vi "NATS Async Monitor.vi"(6 "stop":refnum<notifier>, 8 "error in":errorcluster, 9 "message queue":refnum<queue>, 10 "request queue":refnum<queue>, 11 "nats connection in":T1={"connection ID"=refnum, "server INFO"="", "timeout ms"=5000, "verbose?"=FALSE, "server headers?"=FALSE, "client headers?"=FALSE}) -> (0 "error out":errorcluster)   [LabVIEW 2023, in "NATS Core.lvlib"]
doc: "Reads a message from the NATS server."
uses:
  NATS Core.lvlib
  Controls/nats connection.ctl
  Controls/request queue.ctl
  Controls/nats message.ctl
  Controls/msg type.ctl
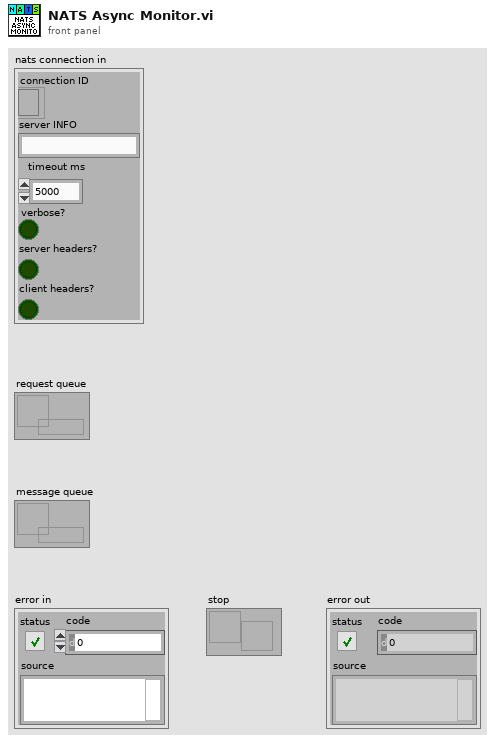
[diagram p1: front panel]
types:
  T1 = typedef "NATS Core.lvlib/nats connection.ctl" = cluster{"connection ID":refnum<k5>, "server INFO":string, "timeout ms":i32, "verbose?":bool, "server headers?":bool, "client headers?":bool}
  T2 = typedef "request queue.ctl" = cluster{"reply subject":string, "request queue":refnum<queue>}
  T3 = typedef "NATS Core.lvlib/nats message.ctl" = cluster{"subject":string, "payload":string, "sub id":string, "reply-to":string, "headers":string, "type":T4, "received":timestamp}
  T4 = typedef "NATS Core.lvlib/msg type.ctl" = enum16{"Undefined", "MSG", "HMSG", "+OK", "PING", "PONG", "-ERR", "INFO"}
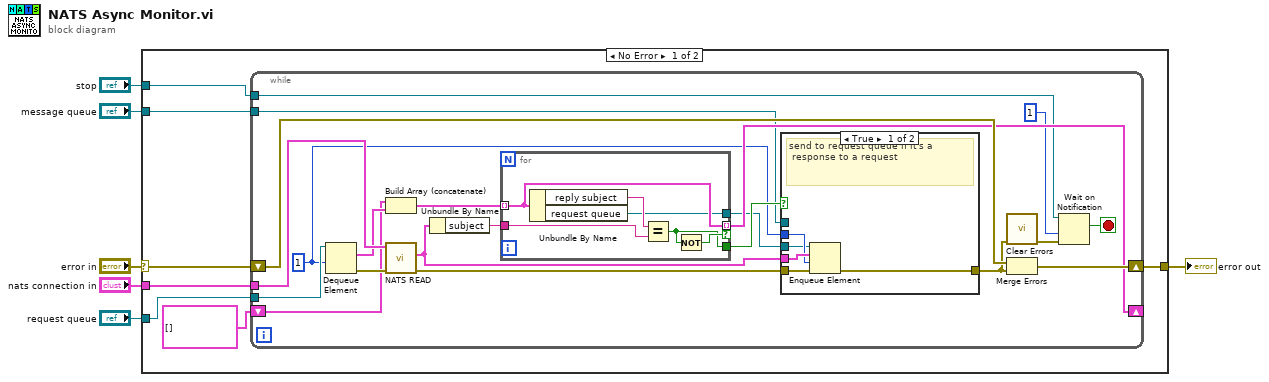
[diagram p0: block diagram]
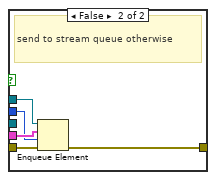
[diagram p2: hidden frame]
diagram:
  n1 = case shown="No Error" "error in" {
    selector: "error in" -> [w12 w51]
    tunnel: "nats connection in" -> [w11 _]
    tunnel: [w13 w51] -> w5
    tunnel: "request queue" -> [w10 _]
    tunnel: "message queue" -> [w8 _]
    tunnel: "stop" -> [w7 _]
    frame No Error {
      n2 = while {
        tunnel: w11 -> [w30]
        tunnel: w10 -> [w29]
        shift-right: [w24] -> _
        shift-left: T2[] [] -> [w27]
        tunnel: w8 -> [w20]
        tunnel: w7 -> [w17]
        shift-right: [w31] -> w13
        shift-left: w12 -> [w32]
        stop <- w16 stop-if-true
        w21 = 1 ("timeout in ms (-1)")
        n3 = Dequeue Element(queue=w29, timeout in ms (-1)=w21) -> (element=w28:T2, error out=w33:errorcluster)  [unwired: 1 in, 2 out]
        n4 = Build Array (concatenate)(w27, w28) -> (w25:T2[])
        n5 = call "NATS READ.vi"("error in"=w33, "nats connection in"=w30) -> ("error out"=w34:errorcluster, "nats message"=w23:T3)  [unwired: 6 in, 2 out]
        n6 = Unbundle By Name(w23) -> ("subject"=w26:string)
        n7 = for {
          tunnel: w25 -> [w48] mode=indexing
          tunnel: w26 -> [w49]
          tunnel: [w48] -> w24 mode=indexing if=w47
          tunnel: [w46] -> w19
          tunnel: [w45] -> w22
          n8 = Unbundle By Name(w48) -> ("reply subject"=w50:string, "request queue"=w46:refnum<queue>)
          n9 = Equal?(x=w50, y=w49) -> (x = y?=w45:bool)
          n10 = Not(x=w45) -> (.not. x?=w47:bool)
        }
        n11 = case shown="True" w22 {
          tunnel: w34 -> [w39 w44]
          tunnel: [w38 w43] -> w15
          tunnel: w23 -> [w37 w42]
          tunnel: w21 -> [w36 w41]
          tunnel: w20 -> [_ w40]
          tunnel: w19 -> [w35 _]
          frame True {
            # "send to request queue if it's a\n response to a request"
            n12 = Enqueue Element(queue=w35, element=w37, timeout in ms (-1)=w36, error in (no error)=w39) -> (error out=w38:errorcluster)  [unwired: 2 out]
          }
          frame False {
            # "send to stream queue otherwise"
            n13 = Enqueue Element(queue=w40, element=w42, timeout in ms (-1)=w41, error in (no error)=w44) -> (error out=w43:errorcluster)  [unwired: 2 out]
          }
        }
        n14 = call <vilib>:"Clear Errors.vi"("error in (no error)"=w15) -> ("error out"=w14:errorcluster)  [unwired: 5 in, 1 out]
        n15 = Merge Errors(w32, w15) -> (w31:errorcluster)
        n16 = Wait on Notification(notifier=w17, timeout in ms (-1)=1, error in (no error)=w14) -> (notification=w16:bool)  [unwired: 1 in, 3 out]
      }
    }
    frame Error {
    }
  }
  "error out" <- w5
